vi "Global.vi"() -> ()   [LabVIEW 2020]
panel:
  in  "复选框":bool
  out "状态读取":T1 {"输出扭矩(小)" format="%#.3f"; "输入扭矩" format="%#.3f"; "输入编码位移" format="%#.3f"; "工装移载位移" format="%#.3f"; "输入移载位移" format="%#.3f"; "输入旋转位移" format="%#.3f"}
  out "传感器读数":T2 {"电缸压力" format="%#.3f"; "Factorysensor" format="%#.3f"; "吸收电流" format="%#.3f"; "输出扭矩(大)" format="%#.3f"; "输出扭矩(小)" format="%#.3f"; "电缸位移" format="%#.3f"; "输入编码位移" format="%#.3f"; "工装移载位移" format="%#.3f"; "输入移载位移" format="%#.3f"; "输入旋转位移" format="%#.3f"}
  in  "追溯码":string
  in  "产品型号":string
  out "初始化":bool
  in  "CODE_ID":string
  in  "右判定长度":i32
  in  "左判定长度":i32
  in  "右工位判定框":T3
  in  "左工位判定框":T3
  in  "右工位判定参数":T4
  in  "左工位判定参数":T5
  in  "当前试验项":enum16{"左工位", "右工位", "完成"}(ring)
  in  "USER_ID":string
  in  "DEVICED_ID":string
  in  "FRE_ID":string
  in  "PRODUCT_ID":string
  in  "上序状态":refnum<vi>
  in  "合格数量":i32
  in  "生产数量":i32
  in  "试验项目":bool[](array[boolean])
  out "模式":u32
  in  "更换产品":refnum<vi>
  in  "提示信息":refnum<vi>
  in  "程序自动":refnum<vi>
  in  "报警图标":refnum<vi>
  in  "程序关闭":bool
  in  "Info":refnum<vi>
  in  "Result":refnum<vi>
  in  "批次":refnum<vi>
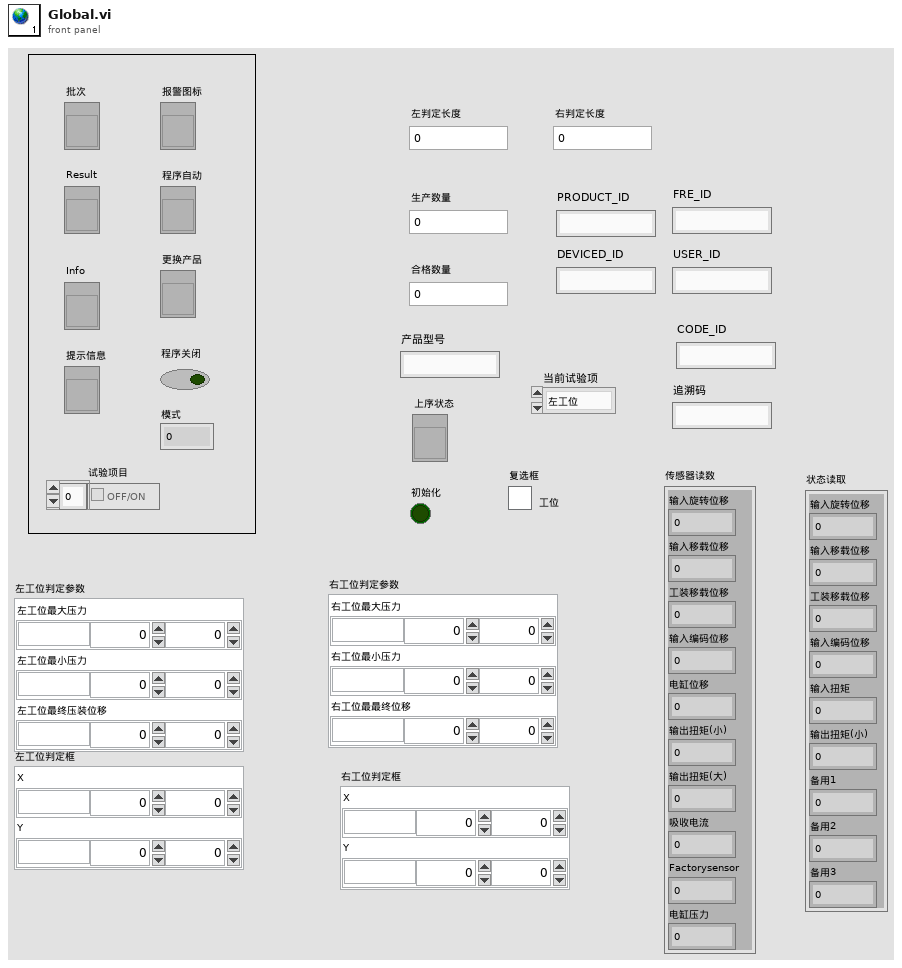
[diagram p1: front panel]
types:
  T1 = cluster{"输入旋转位移":sgl, "输入移载位移":sgl, "工装移载位移":sgl, "输入编码位移":sgl, "输入扭矩":sgl, "输出扭矩(小)":sgl, "备用1":i32, "备用2":i32, "备用3":i32}
  T2 = cluster{"输入旋转位移":sgl, "输入移载位移":sgl, "工装移载位移":sgl, "输入编码位移":sgl, "电缸位移":sgl, "输出扭矩(小)":sgl, "输出扭矩(大)":sgl, "吸收电流":sgl, "Factorysensor":sgl, "电缸压力":sgl}
  T3 = cluster{"X ":cluster{"单位":string, "下限":dbl, "上限":dbl}, "Y":cluster{"单位":string, "下限":dbl, "上限":dbl}}
  T4 = cluster{"右工位最大压力 ":cluster{"单位":string, "下限":dbl, "上限":dbl}, "右工位最小压力":cluster{"单位":string, "下限":dbl, "上限":dbl}, "右工位最最终位移":cluster{"单位":string, "下限":dbl, "上限":dbl}}
  T5 = cluster{"左工位最大压力 ":cluster{"单位":string, "下限":dbl, "上限":dbl}, "左工位最小压力":cluster{"单位":string, "下限":dbl, "上限":dbl}, "左工位最终压装位移":cluster{"单位":string, "下限":dbl, "上限":dbl}}
diagram:
